vi "Reorder Byte Array.vi"(6 "Index In":u32, 7 "InStructure":bool, 8 "Error In":errorcluster, 10 "Byte Stream In":u8[](array[numeric]), 11 "Variant":variant) -> (0 "Error Out":errorcluster, 2 "Byte Stream Out":u8[](array[numeric]), 4 "Index Out":u32)   [LabVIEW 2019, in "TwinCAT ADS.lvlib" / "PLC.lvlib"]
uses:
  <userlib>/PMA/High Level/PLC/PLC.lvlib
  <vilib>/Utility/error.llb/Error Cluster From Error Code.vi
  <vilib>/ErrorRing/Error Ring.xnode
  <vilib>/Utility/Data Type/NI_Data Type.lvlib
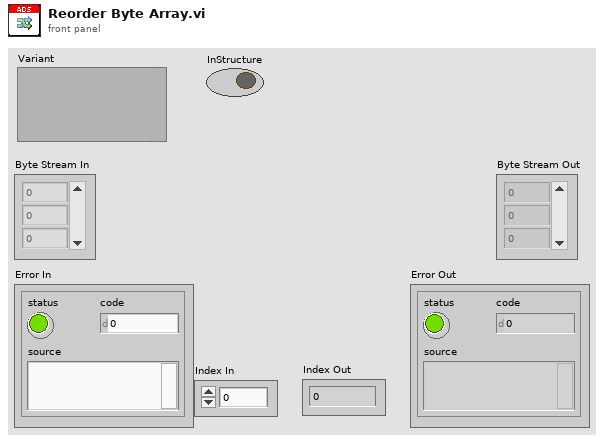
[diagram p1: front panel]
types:
  T1 = typedef "NI_Data Type.lvlib/Data Type.ctl" = enum8{"Invalid Type", "Void", "I8", "I16", "I32", "I64", "U8", "U16", "U32", "U64", "Single Float", "Double Float", "Extended Float", "Single Complex", "Double Complex", "Extended Complex", "Enum U8", "Enum U16", "Enum U32", "Enum U64", "Single Float With Unit", "Double Float With Unit", "Extended Float With Unit", "Single Complex with Unit", "Double Complex with Unit", "Extended Complex with Unit", "Boolean", "String", "Path", "Picture", "Tag", "Array", "Cluster", "Variant", "LV Variant", "Waveform", "Timestamp", "Digital Waveform", "Digital Data", "ExpressData", "Refnum", "External Data", "VI", "Poly VI", "LabVIEW Class Instance", "Fixed Point", "Set Collection", "Map Collection"}
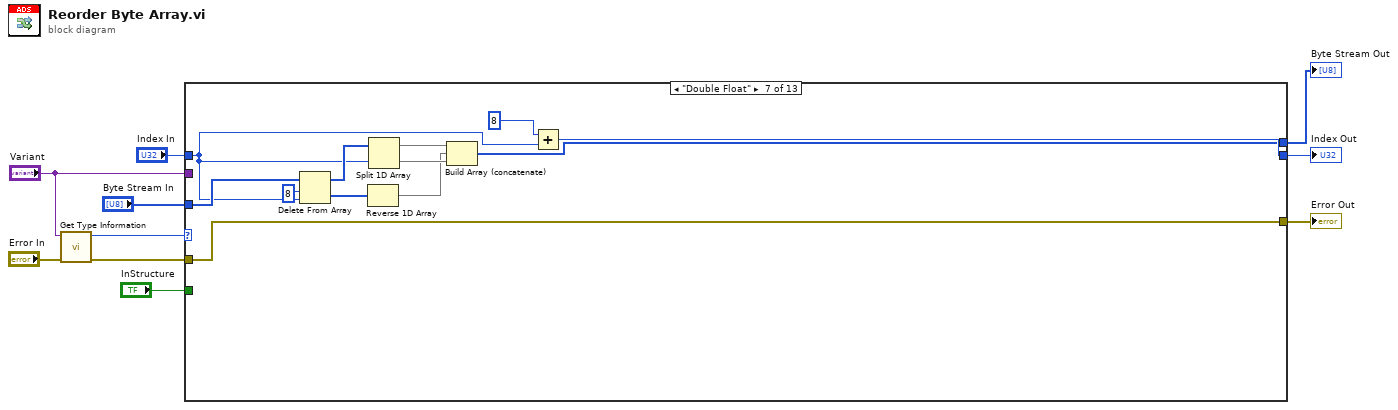
[diagram p0: block diagram]
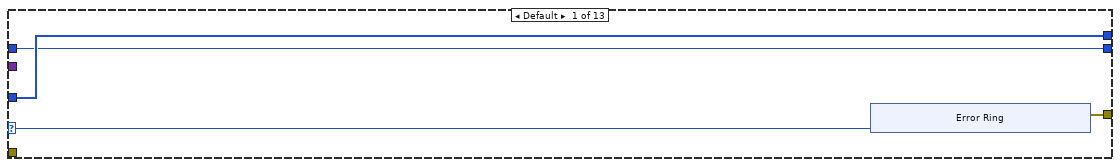
[diagram p2: hidden frame]
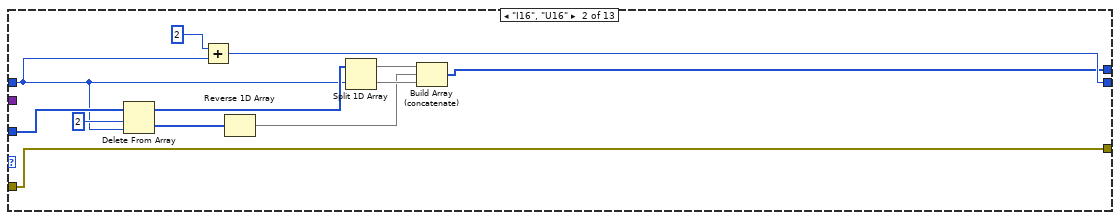
[diagram p3: hidden frame]
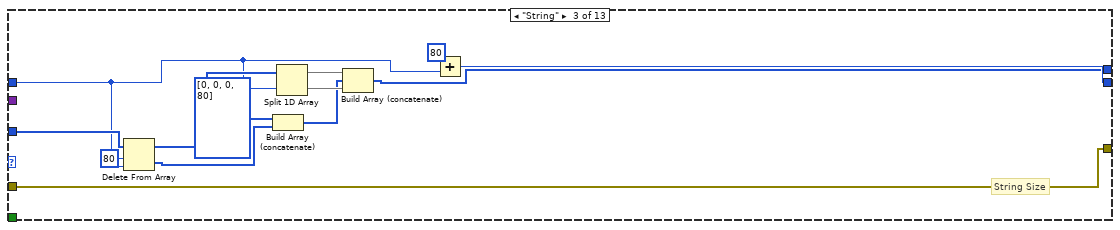
[diagram p4: hidden frame]
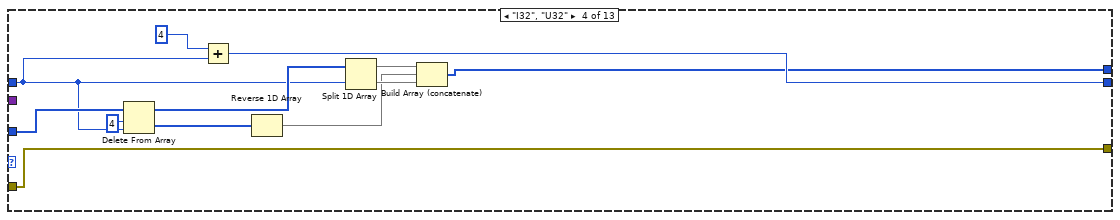
[diagram p5: hidden frame]
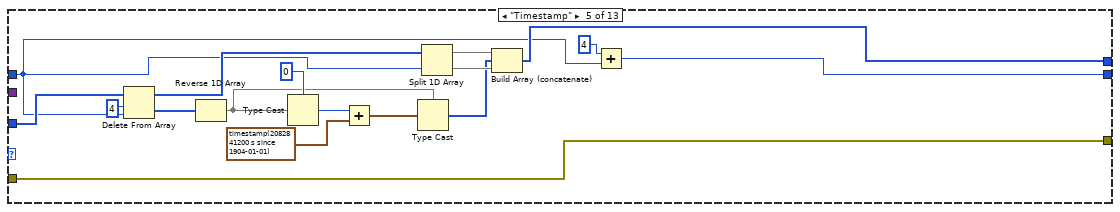
[diagram p6: hidden frame]
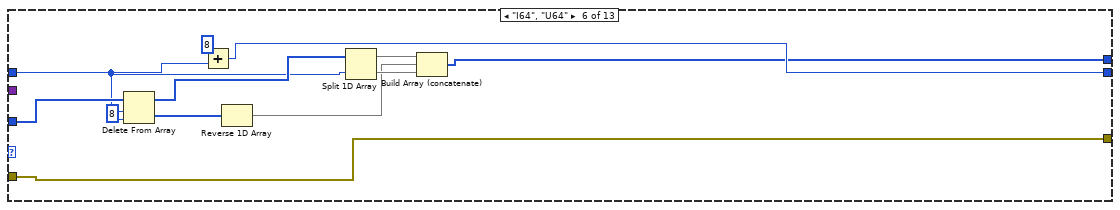
[diagram p7: hidden frame]
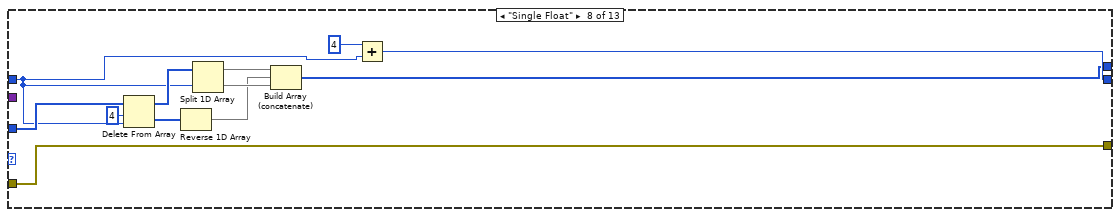
[diagram p8: hidden frame]
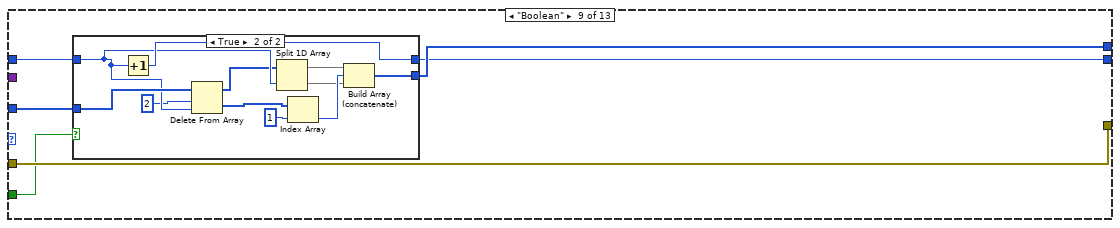
[diagram p9: hidden frame]
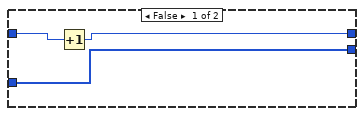
[diagram p10: hidden frame]
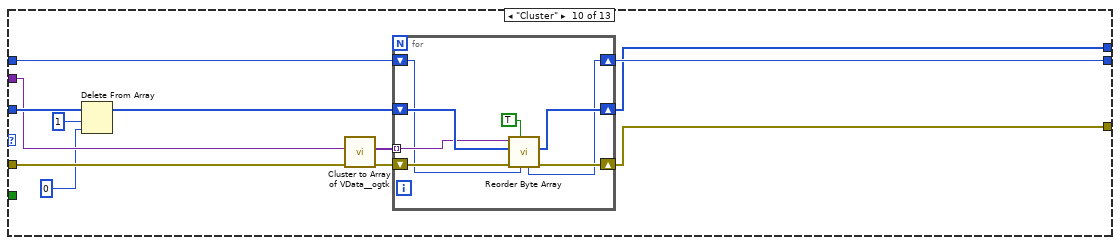
[diagram p11: hidden frame]
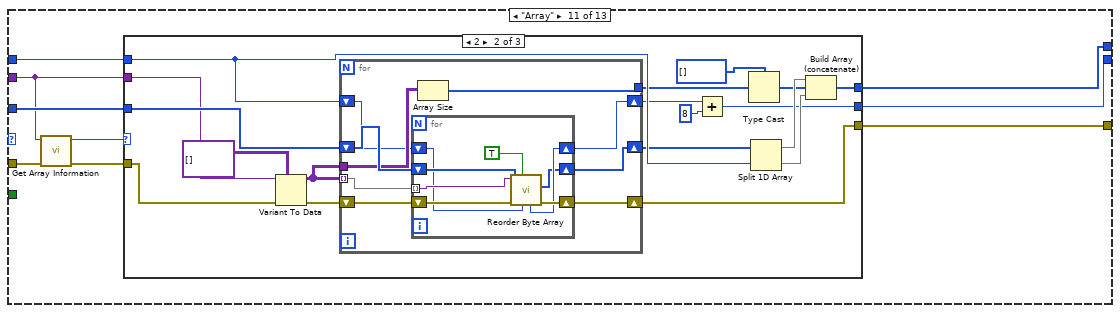
[diagram p12: hidden frame]
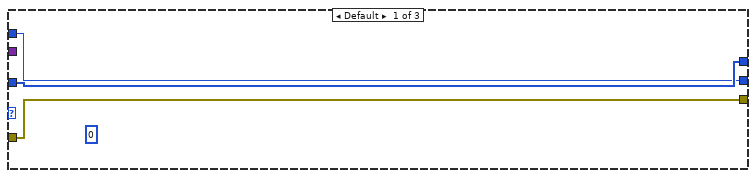
[diagram p13: hidden frame]
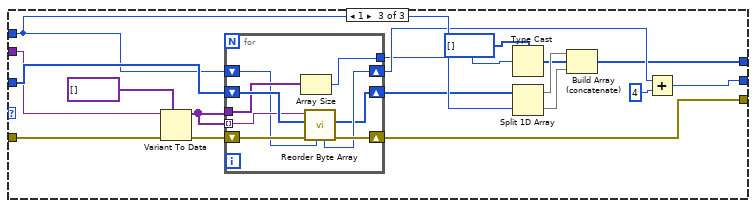
[diagram p14: hidden frame]
diagram:
  n1 = call <vilib>:"Get Type Information.vi"("error in (no error)"="Error In", "variant"="Variant") -> ("error out"=w7:errorcluster, "type"=w9:T1)  [unwired: 5 in, 3 out]
  n2 = case shown="\"Double Float\"" w9 {
    selector: w9 -> [w12 _ _ _ _ _ _ _ _ _ _ _ _]
    tunnel: "Variant" -> [_ _ _ _ _ _ _ _ _ w137 w156 _ _]
    tunnel: w7 -> [_ w33 w46 w58 w75 w87 w99 w111 w114 w141 w155 w228 w231]
    tunnel: [w11 w33 w46 w58 w75 w87 w99 w111 w114 w143 w160 w228 w231] -> w8
    tunnel: "Byte Stream In" -> [w14 w32 w45 w57 w74 w86 w98 w110 w116 w139 w159 w227 w230]
    tunnel: [w14 w27 w40 w52 w69 w81 w93 w105 w117 w136 w152 w227 w230] -> w4
    tunnel: "Index In" -> [w13 w22 w37 w50 w66 w79 w90 w100 w113 w135 w158 w226 w229]
    tunnel: [w13 w31 w44 w56 w73 w85 w97 w109 w115 w138 w157 w226 w229] -> w2
    tunnel: "InStructure" -> [_ _ _ _ _ _ _ _ w112 _ _ _ _]
    frame Default {
      n3 = xnode "Error Ring"("parameter 0"=w12) -> ("error out"=w11:errorcluster)
    }
    frame "I16", "U16" {
      n4 = Delete From Array(array=w32, length=2, index=w22) -> (deleted portion=w24:u8[], array with subset deleted=w29:u8[])
      n5 = Add(x=u32 2, y=w22) -> (x+y=w31:u32)
      n6 = Reverse 1D Array(array=w24) -> (reversed array=w23:u8[])
      n7 = Split 1D Array(array=w29, index=w22) -> (first subarray=w25:u8[], second subarray=w26:u8[])
      n8 = Build Array (concatenate)(w25, w23, w26) -> (w27:u8[])
    }
    frame "String" {
      # "String Size"
      n9 = Delete From Array(array=w45, length=80, index=w37) -> (deleted portion=w39:u8[], array with subset deleted=w42:u8[])
      n10 = Build Array (concatenate)(u8[] [0, 0, 0, 80] ("array"), w39) -> (w35:u8[])
      n11 = Split 1D Array(array=w42, index=w37) -> (first subarray=w36:u8[], second subarray=w38:u8[])
      n12 = Build Array (concatenate)(w36, w35, w38) -> (w40:u8[])
      n13 = Add(x=u32 80, y=w37) -> (x+y=w44:u32)
    }
    frame "I32", "U32" {
      n14 = Delete From Array(array=w57, length=4, index=w50) -> (deleted portion=w48:u8[], array with subset deleted=w54:u8[])
      n15 = Add(x=u32 4, y=w50) -> (x+y=w56:u32)
      n16 = Reverse 1D Array(array=w48) -> (reversed array=w47:u8[])
      n17 = Split 1D Array(array=w54, index=w50) -> (first subarray=w49:u8[], second subarray=w51:u8[])
      n18 = Build Array (concatenate)(w49, w47, w51) -> (w52:u8[])
    }
    frame "Timestamp" {
      n19 = Delete From Array(array=w74, length=4, index=w66) -> (deleted portion=w68:u8[], array with subset deleted=w71:u8[])
      n20 = Reverse 1D Array(array=w68) -> (reversed array=w59:u8[])
      n21 = Type Cast(type=0 ("Time Stamp"), x=w59) -> (*(type *) &x=w61:i32)
      n22 = Add(x=w61, y=timestamp(2082841200 s since 1904-01-01) ("Time Stamp")) -> (x+y=w60:timestamp)
      n23 = Type Cast(type=w59, x=w60) -> (*(type *) &x=w62:u8[])
      n24 = Split 1D Array(array=w71, index=w66) -> (first subarray=w65:u8[], second subarray=w67:u8[])
      n25 = Build Array (concatenate)(w65, w62, w67) -> (w69:u8[])
      n26 = Add(x=u32 4, y=w66) -> (x+y=w73:u32)
    }
    frame "I64", "U64" {
      n27 = Delete From Array(array=w86, length=8, index=w79) -> (deleted portion=w77:u8[], array with subset deleted=w83:u8[])
      n28 = Add(x=u32 8, y=w79) -> (x+y=w85:u32)
      n29 = Reverse 1D Array(array=w77) -> (reversed array=w76:u8[])
      n30 = Split 1D Array(array=w83, index=w79) -> (first subarray=w78:u8[], second subarray=w80:u8[])
      n31 = Build Array (concatenate)(w78, w76, w80) -> (w81:u8[])
    }
    frame "Double Float" {
      n32 = Delete From Array(array=w98, length=8, index=w90) -> (deleted portion=w92:u8[], array with subset deleted=w95:u8[])
      n33 = Reverse 1D Array(array=w92) -> (reversed array=w88:u8[])
      n34 = Split 1D Array(array=w95, index=w90) -> (first subarray=w89:u8[], second subarray=w91:u8[])
      n35 = Build Array (concatenate)(w89, w88, w91) -> (w93:u8[])
      n36 = Add(x=u32 8, y=w90) -> (x+y=w97:u32)
    }
    frame "Single Float" {
      n37 = Delete From Array(array=w110, length=4, index=w100) -> (deleted portion=w102:u8[], array with subset deleted=w107:u8[])
      n38 = Reverse 1D Array(array=w102) -> (reversed array=w101:u8[])
      n39 = Split 1D Array(array=w107, index=w100) -> (first subarray=w103:u8[], second subarray=w104:u8[])
      n40 = Build Array (concatenate)(w103, w101, w104) -> (w105:u8[])
      n41 = Add(x=u32 4, y=w100) -> (x+y=w109:u32)
    }
    frame "Boolean" {
      n42 = case shown="True" w112 {
        tunnel: [w118 w131] -> w117
        tunnel: w116 -> [w118 w130]
        tunnel: [w119 w129] -> w115
        tunnel: w113 -> [w120 w128]
        frame False {
          n43 = Increment(x=w120) -> (x+1=w119:u32)
        }
        frame True {
          n44 = Increment(x=w128) -> (x+1=w129:u32)
          n45 = Delete From Array(array=w130, length=2 ("index"), index=w128) -> (deleted portion=w127:u8[], array with subset deleted=w123:u8[])
          n46 = Split 1D Array(array=w123, index=w128) -> (first subarray=w121:u8[], second subarray=w122:u8[])
          n47 = Index Array(array=w127, index=1) -> (element=w126:u8)
          n48 = Build Array (concatenate)(w121, w126, w122) -> (w131:u8[])
        }
      }
    }
    frame "Cluster" {
      n49 = Delete From Array(array=w139, length=1, index=0) -> (array with subset deleted=w134:u8[])  [unwired: 1 out]
      n50 = call <userlib>:"Cluster to Array of VData__ogtk.vi"("error in (no error)"=w141, "Cluster"=w137) -> ("error out"=w140:errorcluster, "Array of VData"=w142:variant[])  [unwired: 8 in]
      n51 = for {
        shift-right: [w148] -> w143
        shift-left: w140 -> [w147]
        tunnel: w142 -> [w150] mode=indexing
        shift-right: [w149] -> w136
        shift-left: w134 -> [w151]
        shift-right: [w145] -> w138
        shift-left: w135 -> [w144]
        n52 = call <userlib>:"Reorder Byte Array.vi"("Index In"=w144, "InStructure"=TRUE, "Error In"=w147, "Byte Stream In"=w151, "Variant"=w150) -> ("Error Out"=w148:errorcluster, "Byte Stream Out"=w149:u8[], "Index Out"=w145:u32)  [unwired: 4 in]
      }
    }
    frame "Array" {
      n53 = call <vilib>:"Get Array Information.vi"("error in (no error)"=w155, "variant"=w156) -> ("error out"=w154:errorcluster, "number of dimensions"=w153:i32)  [unwired: 6 in, 2 out]
      n54 = case shown="2" w153 {
        tunnel: [w162 w181 w216] -> w160
        tunnel: w159 -> [w163 w180 w215]
        tunnel: [w163 w167 w202] -> w152
        tunnel: w158 -> [w161 w179 w214]
        tunnel: [w161 w165 w200] -> w157
        tunnel: w156 -> [_ w175 w210]
        tunnel: w154 -> [w162 w174 w209]
        frame Default {
          (unwired) 0
        }
        frame 2 {
          n55 = Variant To Data(error in=w174, type=variant[][] [], Variant=w175) -> (data=w173:variant[][], error out=w176:errorcluster)
          n56 = for {
            shift-right: [w188] -> w181
            shift-left: w176 -> [w187]
            tunnel: w173 -> [w189] mode=indexing
            shift-right: [w182] -> w166
            shift-left: w180 -> [w190]
            shift-right: [w186] -> w178
            shift-left: w179 -> [w184]
            tunnel: w173 -> [w185]
            tunnel: [w183] -> w172
            n57 = for {
              tunnel: w189 -> [w197] mode=indexing
              shift-right: [w196] -> w188
              shift-left: w187 -> [w195]
              shift-right: [w193] -> w186
              shift-left: w184 -> [w194]
              shift-right: [w192] -> w182
              shift-left: w190 -> [w198]
              n58 = call <userlib>:"Reorder Byte Array.vi"("Index In"=w194, "InStructure"=TRUE, "Error In"=w195, "Byte Stream In"=w198, "Variant"=w197) -> ("Error Out"=w196:errorcluster, "Byte Stream Out"=w192:u8[], "Index Out"=w193:u32)  [unwired: 4 in]
            }
            n59 = Array Size(array=w185) -> (size(s)=w183:i32[])
          }
          n60 = Add(x=w178, y=u32 8) -> (x+y=w165:u32)
          n61 = Type Cast(type=u8[] [] ("Numeric"), x=w172) -> (*(type *) &x=w168:u8[])
          n62 = Split 1D Array(array=w166, index=w179) -> (first subarray=w169:u8[], second subarray=w170:u8[])
          n63 = Build Array (concatenate)(w169, w168, w170) -> (w167:u8[])
        }
        frame 1 {
          n64 = Variant To Data(error in=w209, type=variant[] [], Variant=w210) -> (data=w208:variant[], error out=w211:errorcluster)
          n65 = for {
            shift-right: [w223] -> w216
            shift-left: w211 -> [w222]
            tunnel: w208 -> [w224] mode=indexing
            shift-right: [w217] -> w201
            shift-left: w215 -> [w225]
            shift-right: [w221] -> w213
            shift-left: w214 -> [w219]
            tunnel: w208 -> [w220]
            tunnel: [w218] -> w207
            n66 = Array Size(array=w220) -> (size(s)=w218:i32)
            n67 = call <userlib>:"Reorder Byte Array.vi"("Index In"=w219, "Error In"=w222, "Byte Stream In"=w225, "Variant"=w224) -> ("Error Out"=w223:errorcluster, "Byte Stream Out"=w217:u8[], "Index Out"=w221:u32)  [unwired: 5 in]
          }
          n68 = Type Cast(type=u8[] [] ("Numeric"), x=w207) -> (*(type *) &x=w203:u8[])
          n69 = Split 1D Array(array=w201, index=w214) -> (first subarray=w204:u8[], second subarray=w205:u8[])
          n70 = Build Array (concatenate)(w204, w203, w205) -> (w202:u8[])
          n71 = Add(x=w213, y=u32 4) -> (x+y=w200:u32)
        }
      }
    }
    frame "Variant" {
    }
    frame "Void" {
    }
  }
  "Byte Stream Out" <- w4
  "Error Out" <- w8
  "Index Out" <- w2
